vi "UnscentedKalmanFilter_Predict.vi"(5 "f_Func":T1, 7 "F_Func_ExtraData":variant, 9 "dT_Seconds":dbl, 10 "U":T2, 11 "in UnscentedKalmanFiilter":T3) -> (0 "Error":bool, 3 "out UnscentedKalmanFiilter":T3)   [LabVIEW 2019, in "Trajectory_Library.lvlib"]
doc: "Project the model into the future with a new control input u.\n \nInputs:\n - inUnscentedKalmanFilter -- filter data cluster\n - u -- New control input from controller.\n - dtSeconds -- Timestep for prediction.\n - F_Func -- function reference. A vector-valued function of x and u that returns the measurement vector\n - F_FuncExtra -- extra data, if any, for F_Func\n\nOutputs:\n - outUnscentedKalmanFilter -- updated filter data cluster\n - error -- If TRUE, an error occured."
uses:
  Trajectory_Library.lvlib
  UNSCENTED_KALMAN_FILTER.ctl
  <vilib>/Analysis/Matrix/Datatypes/RealMatrix.ctl
  MERWE_SCALED_SIGMA_PTS.ctl
  BiFun_Matrix_FUNC_TYPE.ctl
  MatBuilder_Create.vi
  <vilib>/Analysis/7linalg.llb/Transpose Matrix.vi
  <vilib>/Analysis/7linalg.llb/Real Transpose Matrix.vi
  <vilib>/Analysis/baseanly.llb/A x B.vi
  <vilib>/Analysis/baseanly.llb/Real A x B.vi
  Discretization_DiscretizeA.vi
  <vilib>/Analysis/Matrix/Numeric/Add/Add - RM,RM.vi
  <vilib>/Analysis/Matrix/Numeric/Multiply/Multiply.vi
  <vilib>/Analysis/Matrix/Numeric/Multiply/Multiply - RM,R.vi
  Matrix_Exp.vi
  <vilib>/Analysis/Matrix/NI_Matrix.lvlib
panel:
  # "State Estimate <Statess,1>"
  # "<States, States>"
  # "<States, ?>"
  # "<Statess,  States>"
  # "<Outputs, Outputs>"
  # "<?, 1>"
  # "<?, 1>"
  # "State Estimate <Statess,1>"
  # "<States, States>"
  # "<States, ?>"
  # "<Statess,  States>"
  # "<Outputs, Outputs>"
  # "<?, 1>"
  # "<?, 1>"
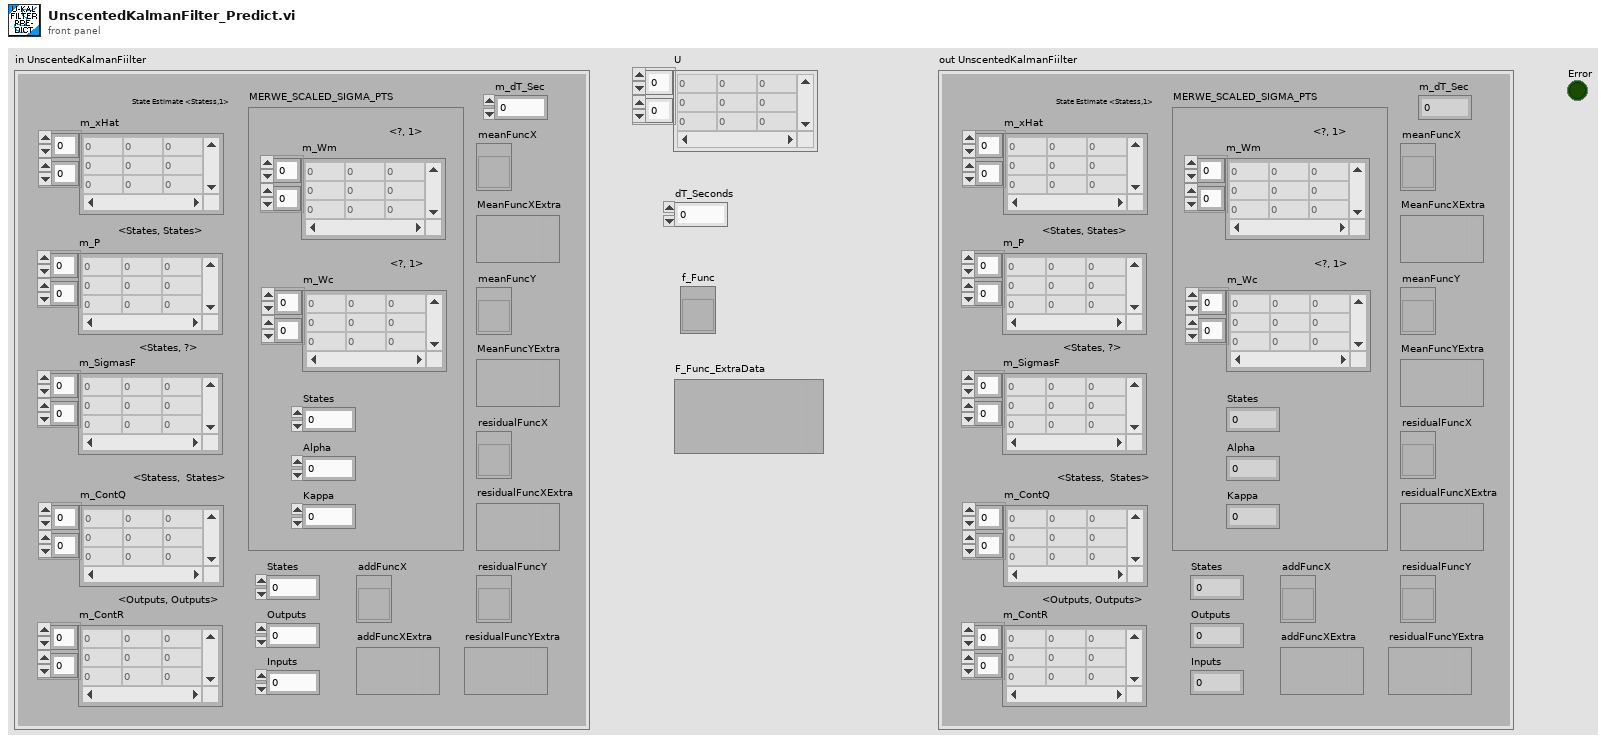
[diagram p1: front panel]
types:
  T1 = typedef "Trajectory_Library.lvlib/BiFun_Matrix_FUNC_TYPE.ctl" = refnum<vi>
  T2 = typedef "NI_Matrix.lvlib/RealMatrix.ctl" = dbl[][]
  T3 = typedef "Trajectory_Library.lvlib/UNSCENTED_KALMAN_FILTER.ctl" = cluster{"m_P":T2, "m_xHat":T2, "States":i32, "Outputs":i32, "m_ContR":T2, "m_ContQ":T2, "m_SigmasF":T2, "m_dT_Sec":dbl, "MERWE_SCALED_SIGMA_PTS":T4, "meanFuncX":T1, "meanFuncY":T1, "residualFuncX":T1, "residualFuncY":T1, "addFuncX":T1, "addFuncXExtra":variant, "residualFuncYExtra":variant, "residualFuncXExtra":variant, "MeanFuncYExtra":variant, "MeanFuncXExtra":variant, "Inputs":i32}
  T4 = typedef "Trajectory_Library.lvlib/MERWE_SCALED_SIGMA_PTS.ctl" = cluster{"m_Wm":T2, "States":i32, "Alpha":dbl, "m_Wc":T2, "Kappa":i32}
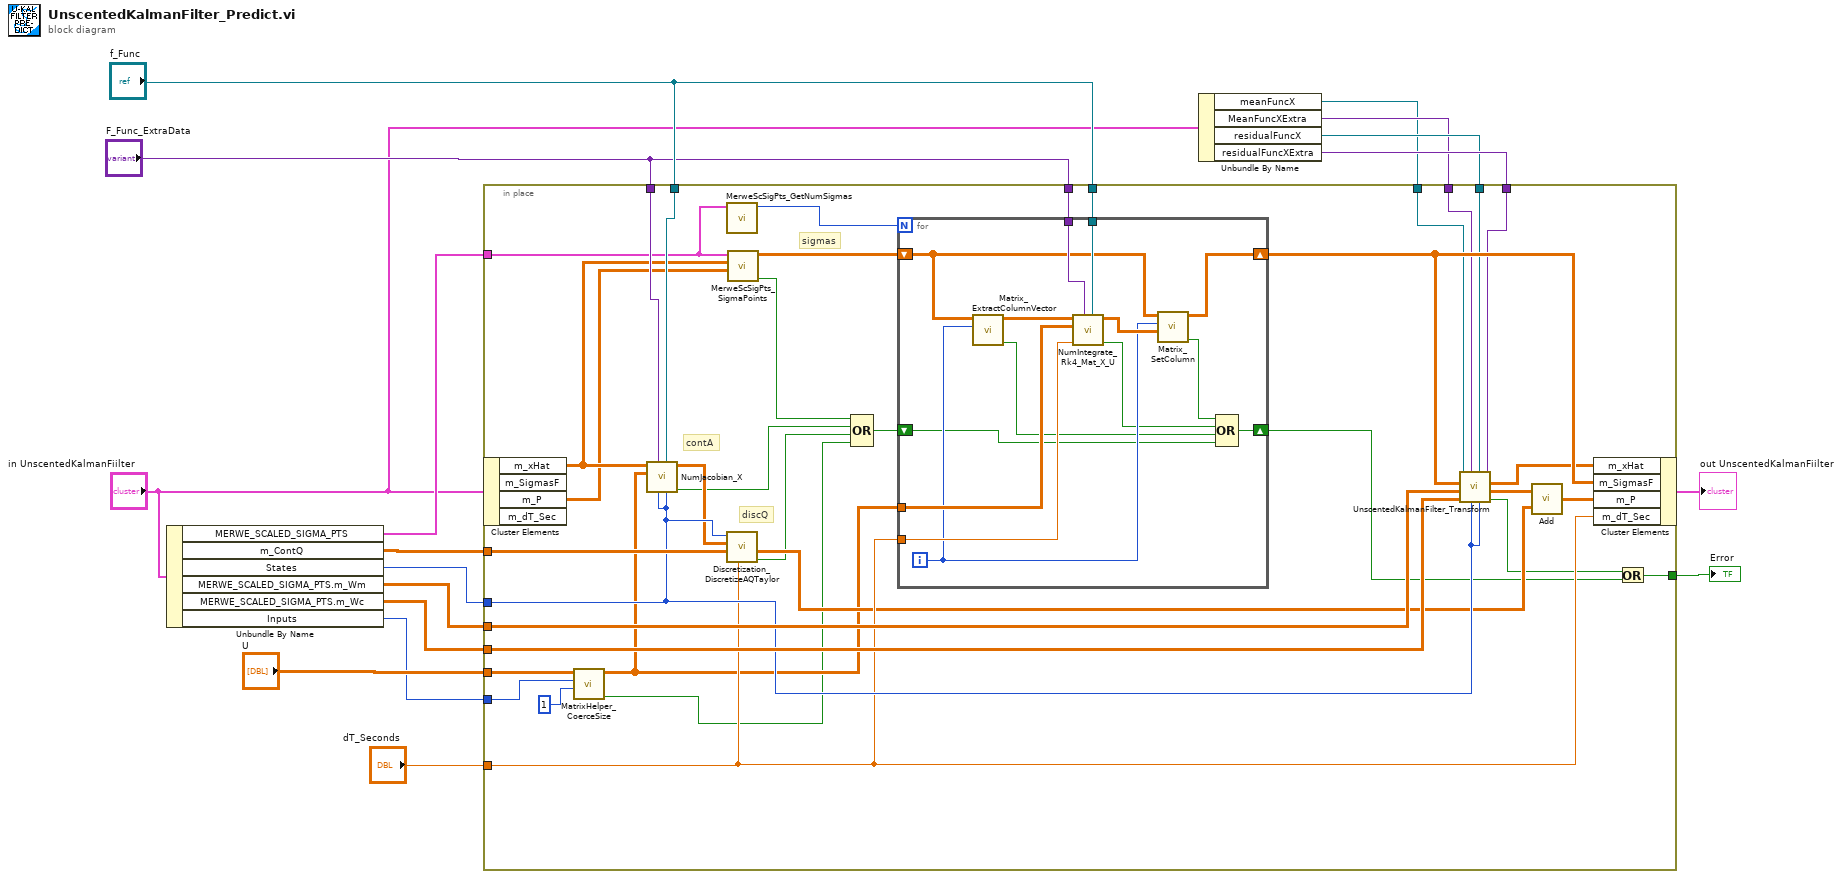
[diagram p0: block diagram]
diagram:
  n1 = Unbundle By Name("in UnscentedKalmanFiilter") -> ("MERWE_SCALED_SIGMA_PTS"=w8:T4, "m_ContQ"=w15:T2, "States"=w13:i32, "MERWE_SCALED_SIGMA_PTS.m_Wm"=w12:T2, "MERWE_SCALED_SIGMA_PTS.m_Wc"=w11:T2, "Inputs"=w1:i32)
  n2 = Unbundle By Name("in UnscentedKalmanFiilter") -> ("meanFuncX"=w3:T1, "MeanFuncXExtra"=w4:variant, "residualFuncX"=w5:T1, "residualFuncXExtra"=w6:variant)
  n3 = in-place {
    in-place-border: "dT_Seconds" -> [w43]
    in-place-border: w15 -> [w53]
    in-place-border: "f_Func" -> [w52]
    in-place-border: "F_Func_ExtraData" -> [w51]
    in-place-border: "U" -> [w21]
    in-place-border: w13 -> [w45]
    in-place-border: w12 -> [w49]
    in-place-border: w11 -> [w48]
    in-place-border: "f_Func" -> [w47]
    in-place-border: "F_Func_ExtraData" -> [w46]
    in-place-border: w8 -> [w32]
    in-place-border: w6 -> [w29]
    in-place-border: w5 -> [w28]
    in-place-border: w4 -> [w27]
    in-place-border: w3 -> [w26]
    in-place-border: [w23] -> w2
    in-place-border: w1 -> [w19]
    # "sigmas"
    # "discQ"
    # "contA"
    n4 = in-place-cluster #1("in UnscentedKalmanFiilter") -> ("m_xHat"=w35:T2, "m_P"=w34:T2)  [unwired: 2 out]
    n5 = call "MatrixHelper_CoerceSize.vi"("Columns"=1, "Rows"=w19, "input matrix"=w21) -> ("Coerced"=w18:bool, "output matrix"=w20:T2)  [unwired: 7 in]
    n6 = call "NumJacobian_X.vi"("States"=w45, "F_FUNC"=w47, "Rows"=w45, "ExtraPassedData"=w46, "U"=w20, "X"=w35) -> ("Error"=w37:bool, "Result"=w44:T2)  [unwired: 4 in]
    n7 = call "MerweScSigPts_GetNumSigmas.vi"("MerweScaledSigmaPts"=w32) -> ("NumSigmas"=w33:i32)  [unwired: 10 in]
    n8 = call "Discretization_DiscretizeAQTaylor.vi"("dT_Seconds"=w43, "ContQ"=w53, "ContA"=w44, "States"=w45) -> ("Error"=w38:bool, "DiscQ"=w40:T2)  [unwired: 5 in, 1 out]
    n9 = call "MerweScSigPts_SigmaPoints.vi"("P"=w34, "X"=w35, "MerweScaledSigmaPts"=w32) -> ("Error"=w31:bool, "SigmaPoints"=w36:T2)  [unwired: 7 in]
    n10 = Compound Arithmetic op=OR(w31, w37, w38, w18) -> (w39:bool)
    n11 = for {
      N: w33 -> [_]
      tunnel: w52 -> [w67]
      tunnel: w51 -> [w66]
      tunnel: w20 -> [w65]
      tunnel: w43 -> [w64]
      shift-right: [w62] -> w50
      shift-left: w36 -> [w57]
      shift-right: [w59] -> w24
      shift-left: w39 -> [w58]
      i -> [w60]
      n12 = call "Matrix_ExtractColumnVector.vi"("Column"=w60, "input matrix"=w57) -> ("Error"=w54:bool, "output column"=w63:T2)  [unwired: 8 in]
      n13 = call "NumIntegrate_Rk4_Mat_X_U.vi"("NumInt_RK4_Func_Type"=w67, "PassedData"=w66, "dT_Seconds"=w64, "U"=w65, "X"=w63) -> ("Error"=w55:bool, "OUTPUT"=w61:T2)  [unwired: 5 in]
      n14 = call "Matrix_SetColumn.vi"("Fill Vector"=w61, "Column"=w60, "input matrix"=w57) -> ("Error"=w56:bool, "output matrix"=w62:T2)  [unwired: 7 in]
      n15 = Compound Arithmetic op=OR(w56, w55, w54, w58) -> (w59:bool)
    }
    n16 = call "UnscentedKalmanFilter_Transform.vi"("ResidualFuncExtra"=w29, "Dim"=w45, "residualFunc"=w28, "S"=w45, "MeanFuncExtra"=w27, "Wc"=w48, "Wm"=w49, "Sigmas"=w50, "MeanFunc"=w26) -> ("Error"=w25:bool, "P"=w41:T2, "X"=w30:T2)
    n17 = call-poly <vilib>:"Add.vi"("Real Matrix B"=w40, "Real Matrix A"=w41) -> ("A + B"=w42:T2)
    n18 = in-place-cluster #1("m_xHat"=w30, "m_SigmasF"=w50, "m_P"=w42, "m_dT_Sec"=w43) -> (→"out UnscentedKalmanFiilter":T3)
    n19 = Or(x=w25, y=w24) -> (x .or. y?=w23:bool)
  }
  "Error" <- w2
